vi "DLL 호출.vi"() -> ()   [LabVIEW 2014]
panel:
  in  "n":i32
  out "웨이브폼 그래프":dbl[](graph)
  out "array":dbl[](array[numeric])
  in  "경로":path
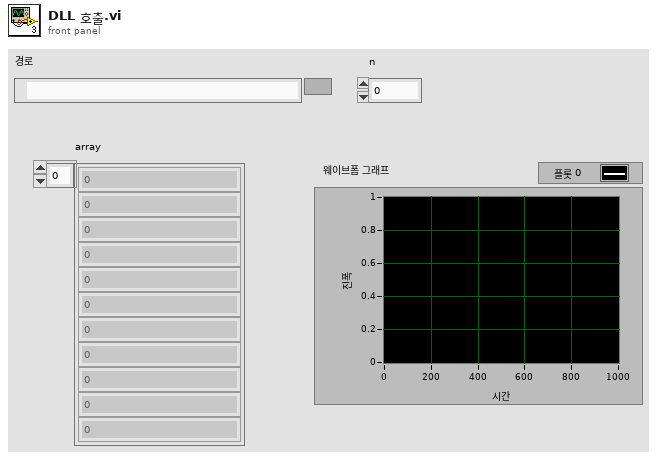
[diagram p1: front panel]
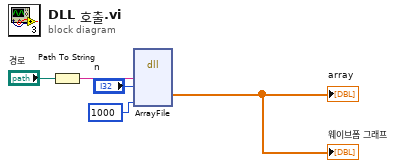
[diagram p0: block diagram]
diagram:
  n1 = Path To String(path="경로") -> (string=w4:string)
  n2 = dll-call lib="PTH2]abs CUsersLVEDU09\tDocumentsYSKbuild공유라이브러리만들기\nSharedLib.dll" fn="ArrayFile"("filePath"=w4, "n"="n", "len"=1000) -> ("array"=→"array" →"웨이브폼 그래프":dbl[])  [unwired: 8 in, 2 out]
